vi "Send.vi"(8 "error in (no error)":errorcluster, 10 "Message":refnum<class "MSG.lvclass">, 11 "DataSocketMessenger in":refnum<class "DataSocketMessenger.lvclass">) -> (0 "error out":errorcluster, 3 "DataSocketMessenger out":refnum<class "DataSocketMessenger.lvclass">)   [LabVIEW 2011, in "Messenging.lvlib" / "DataSocketMessenger.lvclass"]
uses:
  DataSocketMessenger.lvclass
  TextVarientMessage/MSG.lvclass
  DataSocketMessenger.lvclass/DataSocketMessenger.ctl
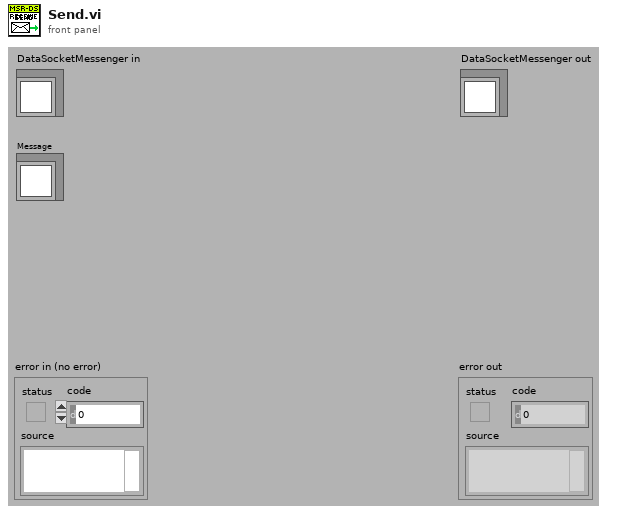
[diagram p1: front panel]
types:
  T1 = enum16{"Read", "Write", "ReadWrite", "BufferedRead", "BufferedReadWrite"}
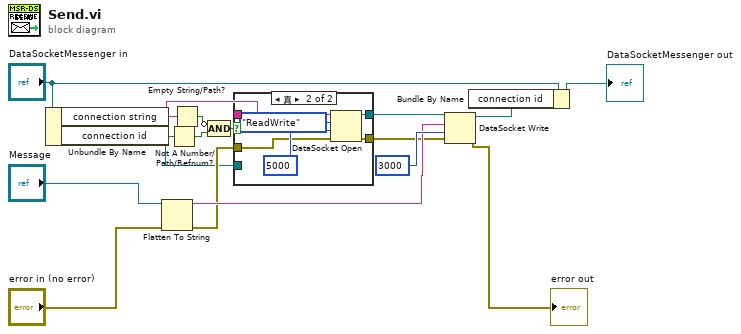
[diagram p0: block diagram]
diagram:
  n1 = Unbundle By Name("DataSocketMessenger in") -> ("connection string"=w6:string, "connection id"=w3:refnum<k13>)
  n2 = Flatten To String(anything="Message", error in (no error)="error in (no error)") -> (data string=w12:string, error out=w5:errorcluster)  [unwired: 3 out]
  n3 = Not A Number/Path/Refnum?(number/path/refnum=w3) -> (NaN/Path/Refnum?=w8:bool)
  n4 = Empty String/Path?(string/path=w6) -> (empty?=w9:bool)
  n5 = Compound Arithmetic op=AND(invert w9, w8) -> (w7:bool)
  n6 = case shown="真" w7 {
    tunnel: [w18 w24] -> w10
    tunnel: w6 -> [_ w23]
    tunnel: w5 -> [w17 w21]
    tunnel: [w17 w20] -> w4
    tunnel: w3 -> [w18 _]
    frame False {
    }
    frame True {
      n7 = DataSocket Open(8:w21, 9:5000 ("ms timeout (10000)"), 10:T1."ReadWrite" ("mode"), 11:w23) -> (0:w20:errorcluster, 3:w24:refnum<k13>)
    }
  }
  n8 = DataSocket Write(8:w4, 9:3000 ("ms timeout (0)"), 10:w12, 11:w10) -> (0:→"error out":errorcluster, 3:w1:refnum<k13>)  [unwired: 1 out]
  n9 = Bundle By Name(cluster="DataSocketMessenger in", "connection id"=w1) -> (→"DataSocketMessenger out":refnum<class "DataSocketMessenger.lvclass">)
